vi "Day 21-Calculate Move and Score.vi"(8 "Dice Roll Sum":u64, 9 "Score in":u64, 11 "Position in":u64) -> (1 "Score out":u64, 3 "Position out":u64)   [LabVIEW 2021]
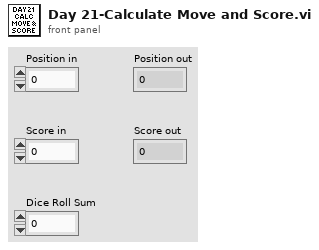
[diagram p1: front panel]
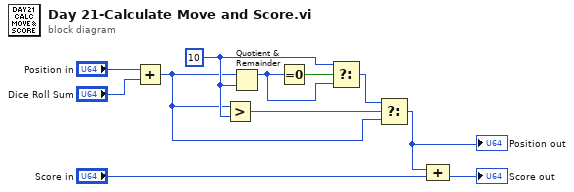
[diagram p0: block diagram]
diagram:
  w11 = u64 10
  n1 = Add(x="Position in", y="Dice Roll Sum") -> (x+y=w5:u64)
  n2 = Greater?(x=w5, y=w11) -> (0:w4:bool)
  n3 = Quotient & Remainder(x=w5, y=w11) -> (x-y*floor(x/y)=w8:u64)  [unwired: 1 out]
  n4 = Equal To 0?(x=w8) -> (x = 0?=w7:bool)
  n5 = Select(t=w11, s=w7, f=w8) -> (s? t:f=w9:u64)
  n6 = Select(t=w9, s=w4, f=w5) -> (s? t:f=w6:u64)
  "Position out" <- w6
  n7 = Compound Arithmetic op=ADD(w6, "Score in") -> (→"Score out":u64)
